vi "Read GUID.vi"(8 "error in (no error)":errorcluster, 11 "Attribute.Identity in":refnum<class "Attribute.Identity.lvclass">) -> (0 "error out":errorcluster, 2 "GUID":string, 3 "Attribute.Identity out":refnum<class "Attribute.Identity.lvclass">)   [LabVIEW 2013, in "Attribute.Identity.lvclass"]
uses:
  Attribute.Identity.lvclass
  Attribute.Identity.lvclass/Attribute.Identity.ctl
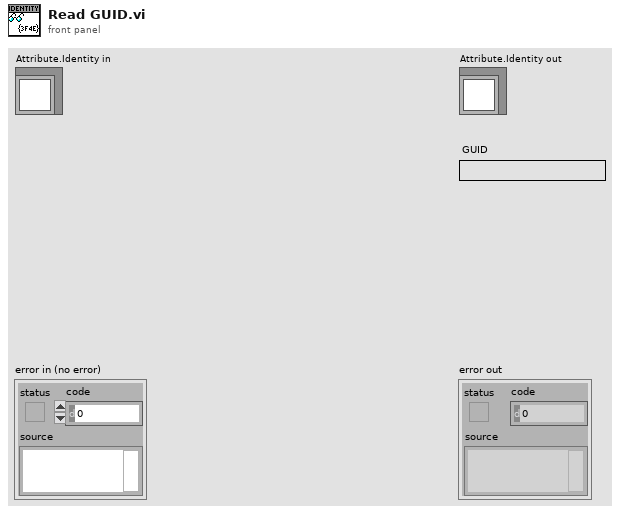
[diagram p1: front panel]
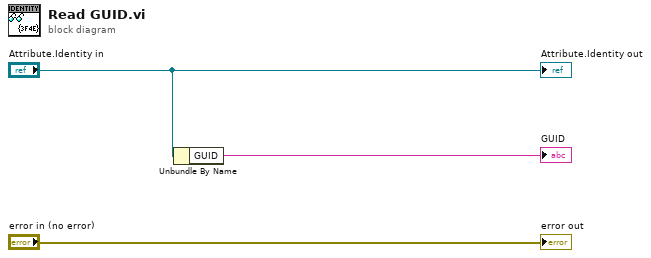
[diagram p0: block diagram]
diagram:
  n1 = Unbundle By Name("Attribute.Identity in") -> ("GUID"=→"GUID":string)
  "error out" <- "error in (no error)"
  "Attribute.Identity out" <- "Attribute.Identity in"
